vi "tcs shm get Sample kernel Target LV.vi"(8 "error in (no error)":errorcluster, 11 "kernel_Target_Ctl":T1) -> (0 "error out":errorcluster, 2 "function return":i32, 3 "kernel_Target_Ctl out":T1)   [LabVIEW 2016, in "SALLV_tcs.lvlib"]
doc: "int tcs_shm_getSample_kernel_TargetLV(tcs_kernel_TargetLV *kernel_Target_Ctl );"
uses:
  SALLV_tcs.lvlib
  SALLV_tcs.so
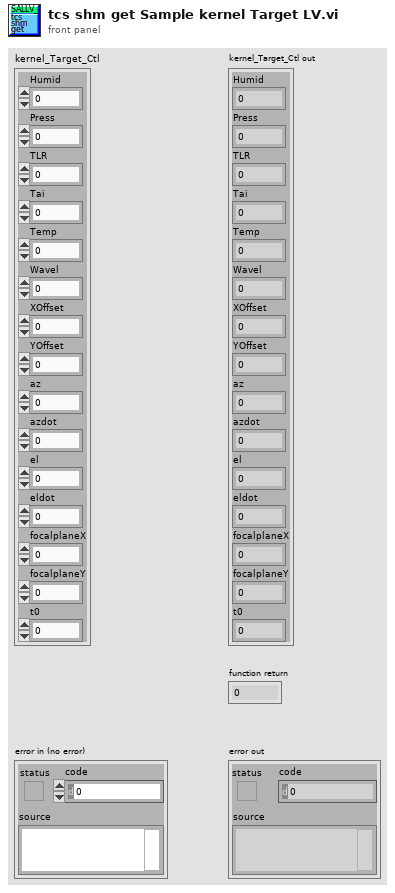
[diagram p1: front panel]
types:
  T1 = cluster{"Humid":sgl, "Press":sgl, "TLR":sgl, "Tai":sgl, "Temp":sgl, "Wavel":sgl, "XOffset":sgl, "YOffset":sgl, "az":sgl, "azdot":sgl, "el":sgl, "eldot":sgl, "focalplaneX":sgl, "focalplaneY":sgl, "t0":sgl}
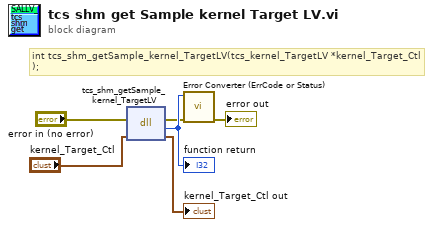
[diagram p0: block diagram]
diagram:
  # "int tcs_shm_getSample_kernel_TargetLV(tcs_kernel_TargetLV *kernel_Target_Ctl );"
  n1 = dll-call lib="home/andres/Desktop/SALLV_tcs/SALLV_tcs.*" fn="tcs_shm_getSample_kernel_TargetLV"(error in="error in (no error)", "kernel_Target_Ctl"="kernel_Target_Ctl") -> (error out=w2:errorcluster, w6:i32, "kernel_Target_Ctl"=→"kernel_Target_Ctl out":T1)  [unwired: 2 in, 1 out]
  "function return" <- w6
  n2 = call "Error Converter (ErrCode or Status).vi"("error in (no error)"=w2, "error code"=w6) -> ("error out"=→"error out":errorcluster)  [unwired: 9 in]
